vi "iXonEMCCD_Initialize.vi"() -> ()   [LabVIEW 2025]
panel:
  out "Initialize success?":bool
  out "DLL error code":u32
  out "error out":errorcluster
  in  "directory (\"\")":string
  in  "error in":errorcluster
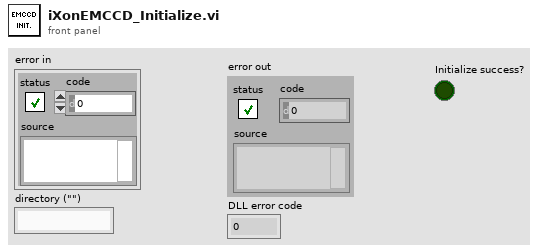
[diagram p1: front panel]
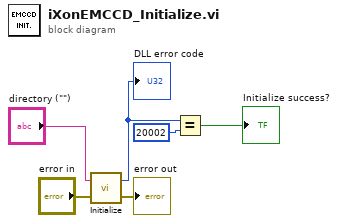
[diagram p0: block diagram]
diagram:
  n1 = call "Initialize.vi"("error in (no error)"="error in", "directory (\"\")"="directory (\"\")") -> ("error out"=→"error out":errorcluster, "DLL error code"=w2:u32)
  "DLL error code" <- w2
  n2 = Equal?(x=w2, y=u32 20002) -> (x = y?=→"Initialize success?":bool)
